vi "CheckDuplicateData.vi"(8 "error in (no error)":errorcluster, 10 "ToCheck in":refnum<data-value>, 11 "Cell in":refnum<class "Cell.lvclass">) -> (0 "error out":errorcluster, 1 "IsDuplicate":bool, 2 "ToCheck out":refnum<data-value>, 3 "Cell out":refnum<class "Cell.lvclass">)   [LabVIEW 2010, in "Cell.lvclass"]
uses:
  Cell.lvclass
  LLNode/LLNode.lvclass
  Cell.lvclass/Cell.ctl
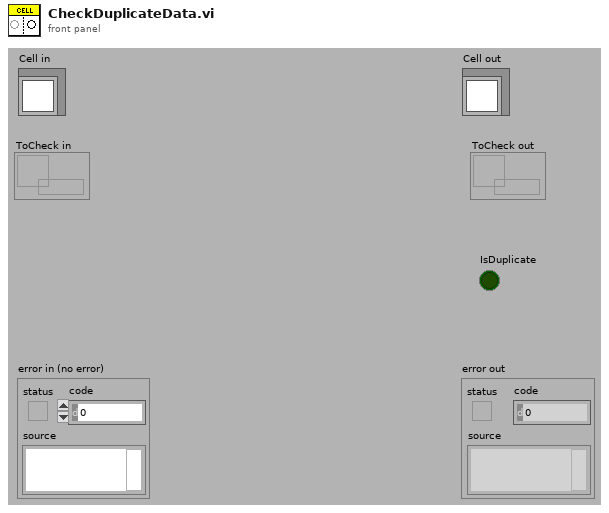
[diagram p1: front panel]
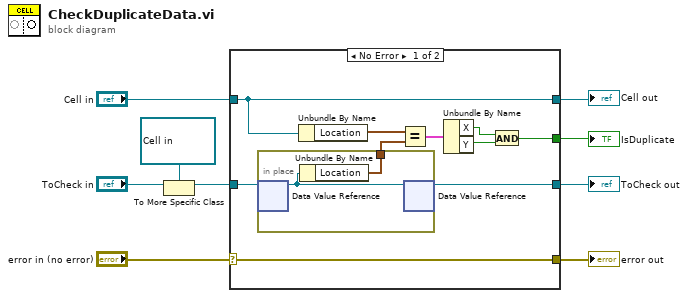
[diagram p0: block diagram]
diagram:
  n1 = To More Specific Class(target class=refnum<data-value> refnum ("data value reference"), reference="ToCheck in") -> (specific class reference=w5:refnum<data-value>)  [unwired: 1 in, 1 out]
  n2 = case shown="No Error" "error in (no error)" {
    selector: "error in (no error)" -> [w10 w22]
    tunnel: "Cell in" -> [w18 w23]
    tunnel: w5 -> [w19 w24]
    tunnel: [w18 w23] -> w4
    tunnel: [w17 w24] -> w3
    tunnel: [w11 _] -> w2
    tunnel: [w10 w22] -> w1
    frame No Error {
      n3 = in-place {
        in-place-border: [w20] -> w15
        n4 = in-place-dvr #1(w19) -> (w21:refnum<class "Cell.lvclass">)  [unwired: 1 out]
        n5 = Unbundle By Name(w21) -> ("Location"=w20:cluster{"X":dbl, "Y":dbl})
        n6 = in-place-dvr #1(w21) -> (w17:refnum<data-value>)  [unwired: 1 out]
      }
      n7 = Unbundle By Name(w18) -> ("Location"=w16:cluster{"X":dbl, "Y":dbl})
      n8 = Equal?(x=w16, y=w15) -> (x = y?=w14:cluster{"X":bool, "Y":bool})
      n9 = Unbundle By Name(w14) -> ("X"=w13:bool, "Y"=w12:bool)
      n10 = And(x=w13, y=w12) -> (x .and. y?=w11:bool)
    }
    frame Error {
    }
  }
  "error out" <- w1
  "Cell out" <- w4
  "ToCheck out" <- w3
  "IsDuplicate" <- w2
